vi "ConfigDlg.vi"(8 "error in (no error)":errorcluster, 11 "ScopePluginsBase in":refnum<class "ScopePluginsBase.lvclass">) -> (0 "error out":errorcluster, 3 "ScopePluginsBase out":refnum<class "ScopePluginsBase.lvclass">)   [LabVIEW 2018, in "ScopePlugins.lvlib" / "ScopePluginsBase.lvclass"]
uses:
  ScopePluginsBase.lvclass
  C:/Program Files (x86)/National Instruments/LabVIEW 2018/user.lib/NIST/BaseClasses/BasePlugin_class/BasePlugin.lvclass
  Shared/TypeDefs/Acquisition.ctl
  Shared/TypeDefs/Trigger.ctl
  Shared/TypeDefs/Channel.ctl
  TypeDefs/InitOptions.ctl
  ScopePluginsBase.lvclass/ScopePluginsBase.ctl
  Shared/TypeDefs/Channels.ctl
  <userlib>/NIST/BaseClasses/BasePlugin_class/BasePlugin.lvclass/BasePlugin.ctl
  Accessors/Read Acquisition.vi
  Accessors/Read Channels.vi
  Accessors/Read Trigger.vi
  <userlib>/NIST/BaseClasses/BasePlugin_class/Accessors/Read PluginIniFilePath.vi
  Accessors/Write Acquisition.vi
  Accessors/Write Trigger.vi
  Accessors/Write Channels.vi
  <vilib>/Utility/config.llb/NI_LVConfig.lvlib
  ScopePlugins.lvlib
panel:
  in  "Trigger Type":T1(tab)
  in  "Input Impedance":u32(ring) items=["1 mega ohm"=0, "50 ohms"=2]
  in  "Maximum Input Frequency":dbl caption="Max. Input Frequency (Hz)" format="%.2f"
  in  "Initialize Options":T2
  out "Actual Sample Rate":dbl=10000000.0 format="%#.2p"
  out "Actual Record Length":i32=1000
  in  "Min Record Length":i32=1000 caption="Min. Record Length"
  in  "Min Sample Rate":dbl=10000000.0 caption="Min. Sample Rate" step=1000000.0 format="%#.2p"
  in  "Enforce Realtime":bool=TRUE
  in  "Vertical Coupling":i32(ring)=1 items=["AC", "DC", "Ground"]
  in  "Probe Attenuation":dbl=1.0 format="%.1f"
  in  "Vertical Offset":dbl caption="Vertical Offset (V)" format="%.2p"
  in  "Vertical Range":dbl=5.0 caption="Vertical Range (V)" format="%.2f"
  in  "Trigger Type 2":T3(tab) caption="Trigger Type"
  in  "Trigger Source":string(combo)="0"
  in  "Trigger Level":dbl format="%.2f"
  in  "Trigger Slope":i32(ring) items=["Positive", "Negative"]
  in  "Coupling":u16(ring)=1 caption="Trigger Coupling" items=["AC"=0, "DC"=1, "HF Reject"=3, "LF Reject"=4, "AC Plus HF Reject"=1001]
  in  "Trigger Slope 2":i32(ring) caption="Trigger Slope" items=["Positive", "Negative"]
  in  "Trigger Source 2":string(combo)="VAL_PFI_1" caption="Trigger Source"
  in  "Coupling 2":u16(ring)=1 caption="Trigger Coupling" items=["AC"=0, "DC"=1, "HF Reject"=3, "LF Reject"=4, "AC Plus HF Reject"=1001]
  in  "High Level":dbl=0.1 caption="Window High Level" format="%.2f"
  in  "Low Level":dbl=-0.1 caption="Window Low Level" format="%.2f"
  in  "Window Mode":i32(ring) items=["Entering", "Leaving"]
  in  "Trigger Source 3":string(combo)="0" caption="Trigger Source"
  in  "Hysteresis":dbl=0.05 format="%.2f"
  in  "Trigger Source 4":string(combo)="0" caption="Trigger Source"
  in  "Trigger Level 2":dbl caption="Trigger Level" format="%.2f"
  in  "Coupling 3":u16(ring)=1 caption="Trigger Coupling" items=["AC"=0, "DC"=1, "HF Reject"=3, "LF Reject"=4, "AC Plus HF Reject"=1001]
  in  "Trigger Slope 3":i32(ring) caption="Trigger Slope" items=["Positive", "Negative"]
  out "Auto Triggered":bool
  in  "Trigger Modifier":i32(ring)=2 items=["None"=1, "Auto Trigger"=2]
  in  "Stop":bool
  in  "Reference Position":dbl=50.0 caption="Ref Position" format="%.1f"
  in  "Trigger Delay":dbl caption="Trigger Delay (s)" format="%#.4p"
  in  "InitOptions":T2
  in  "Save As Button":bool
  in  "Save Button":bool
  in  "Channels":T4[](array[typedef])
  in  "Trigger":T5
  in  "Acquisition":T6={"StartTime"=0.0, "Type"=enum."Normal", "NumPointsMin"=0, "RecordLength"=0, "SampleRate"=0.0, "TimePerRecord"=0.0, "SamplingMode "=enum."Real Time", "Interpolation"=enum."No Interpolation", "NumAverages"=8, "Resolution"=enum."Auto", "EnableAveraging"=FALSE, "Continuous"=FALSE}
  in  "btnCancel":bool
  # "Channel"
  # "Horizontal"
  # "Vertical"
  # "Trigger"
  # "Common Trigger Settings"
  # "Note: When configured for Immediate reference trigger, this example does not configure any additional trigger settings - the acquisition is triggered as soon as possible after being initiated by driver software."
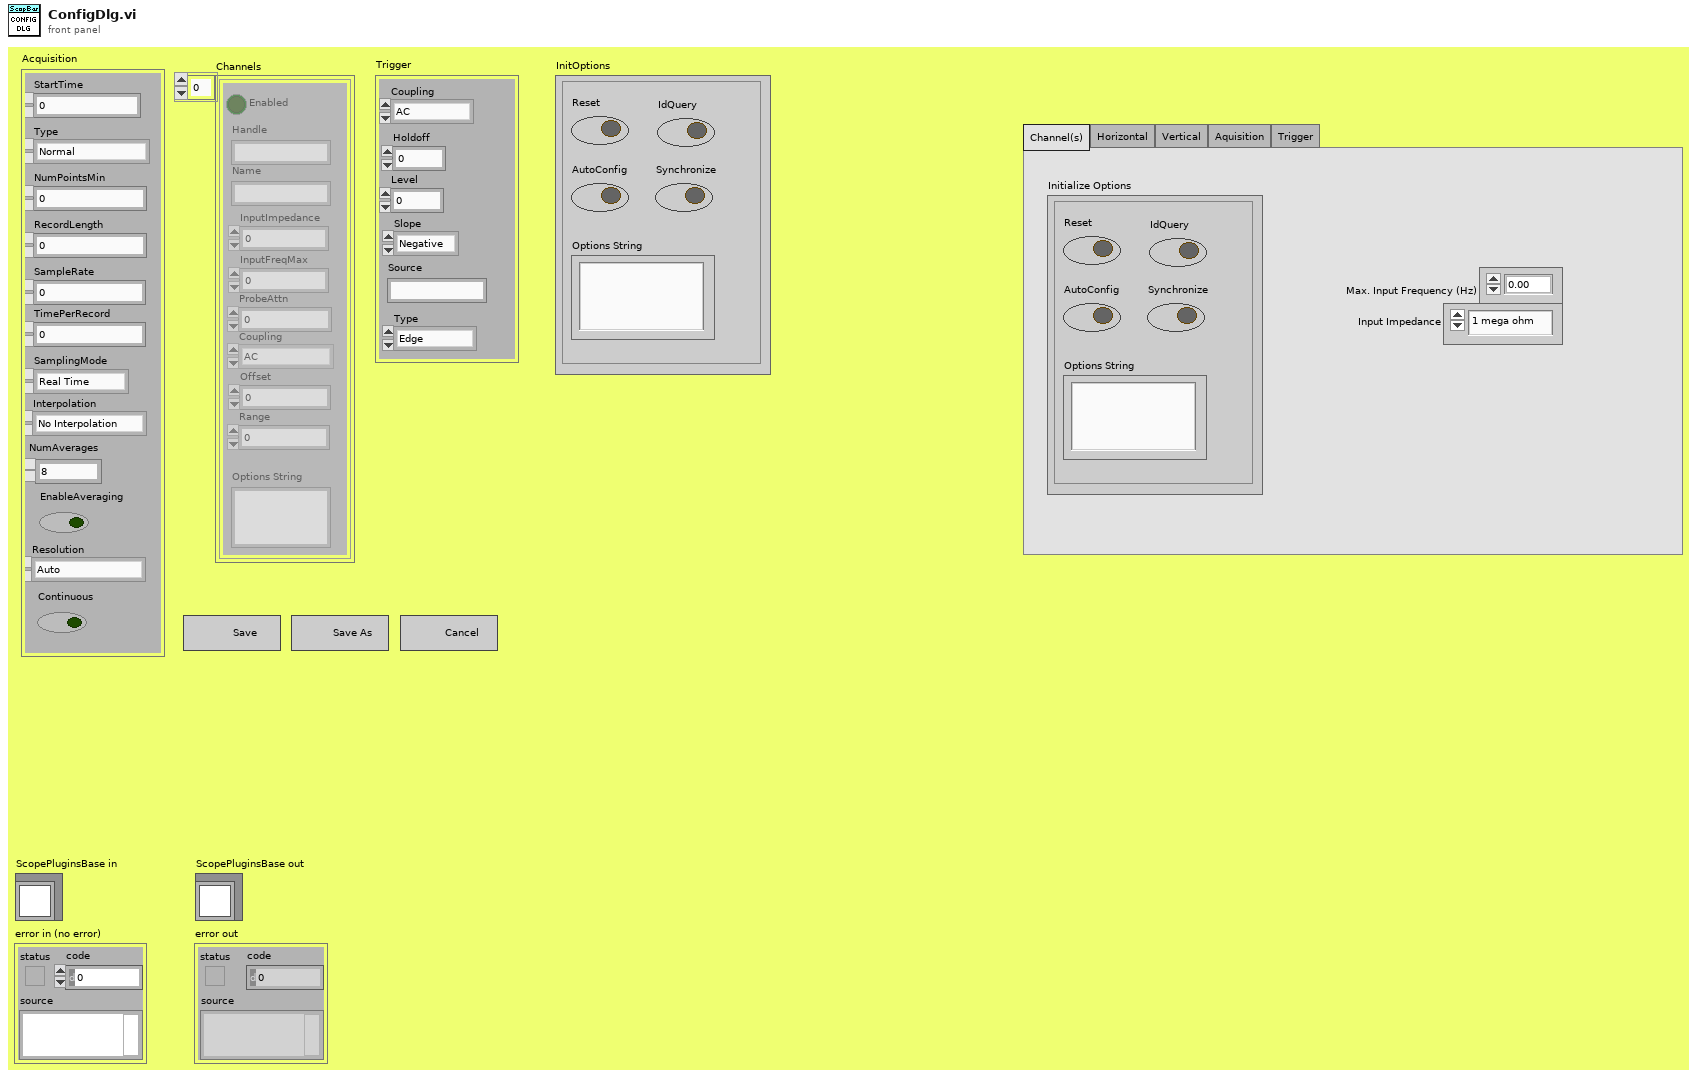
[diagram p1: front panel]
types:
  T1 = enum32{"Channel(s)", "Horizontal", "Vertical", "Aquisition", "Trigger"}
  T2 = typedef "ScopePlugins.lvlib/InitOptions.ctl" = cluster{"Reset":bool, "IdQuery":bool, "AutoConfig":bool, "Options String":string, "Synchronize":bool}
  T3 = enum32{"Immediate", "Edge", "Digital", "Window", "Hysteresis"}
  T4 = typedef "ScopePlugins.lvlib/Channel.ctl" = cluster{"Enabled":bool, "Name":string, "InputImpedance":dbl, "InputFreqMax":dbl, "ProbeAttn":dbl, "Coupling":enum16{"AC", "DC", "GND"}, "Offset":dbl, "Range":dbl, "Handle":string, "Connected":bool, "Options String ":string}
  T5 = typedef "ScopePlugins.lvlib/Trigger.ctl" = cluster{"Coupling":enum16{"AC", "DC", "LF Reject", "HF Reject", "Noise Reject"}, "Holdoff":dbl, "Level":dbl, "Slope":enum16{"Negative", "Positive"}, "Source":string, "Type":enum16{"Edge", "Width", "Runt", "Glitch", "TV", "Immediate", "AC Line"}}
  T6 = typedef "ScopePlugins.lvlib/Acquisition.ctl" = cluster{"StartTime":dbl, "Type":enum16{"Normal", "PeakDetect", "HighRes", "Envelope", "Average"}, "NumPointsMin":i32, "RecordLength":i32, "SampleRate":dbl, "TimePerRecord":dbl, "SamplingMode ":enum16{"Real Time", "Equivalent Time", "Segment", "Real Time Peak Detect", "Real Time High Resolution", "Peak Detect Segment", "High Resolution Segment"}, "Interpolation":enum16{"No Interpolation", "sin(x)/x", "linear", "1 Point sin(x)/x", "2 Point sin(x)/x", "4 Point sin(x)/x", "8 Point sin(x)/x", "16 Point sin(x)/x"}, "NumAverages":i32, "Resolution":enum16{"Auto", "Bits 9", "Bits 10", "Bits 11", "Bits 12"}, "EnableAveraging":bool, "Continuous":bool}
  T7 = enum8{"Enabled", "Disabled", "Disabled and Grayed Out"}
  T8 = enum32{"Invalid", "Default", "Floating", "Floating/Auto-Hide", "Modal"}
  T9 = typedef "ScopePlugins.lvlib/Channels.ctl" = cluster{"Count":i32, "ChannelArray":T4[]}
  T10 = typedef "NI_LVConfig.lvlib/Config Data RefNum.ctl" = refnum<k1>
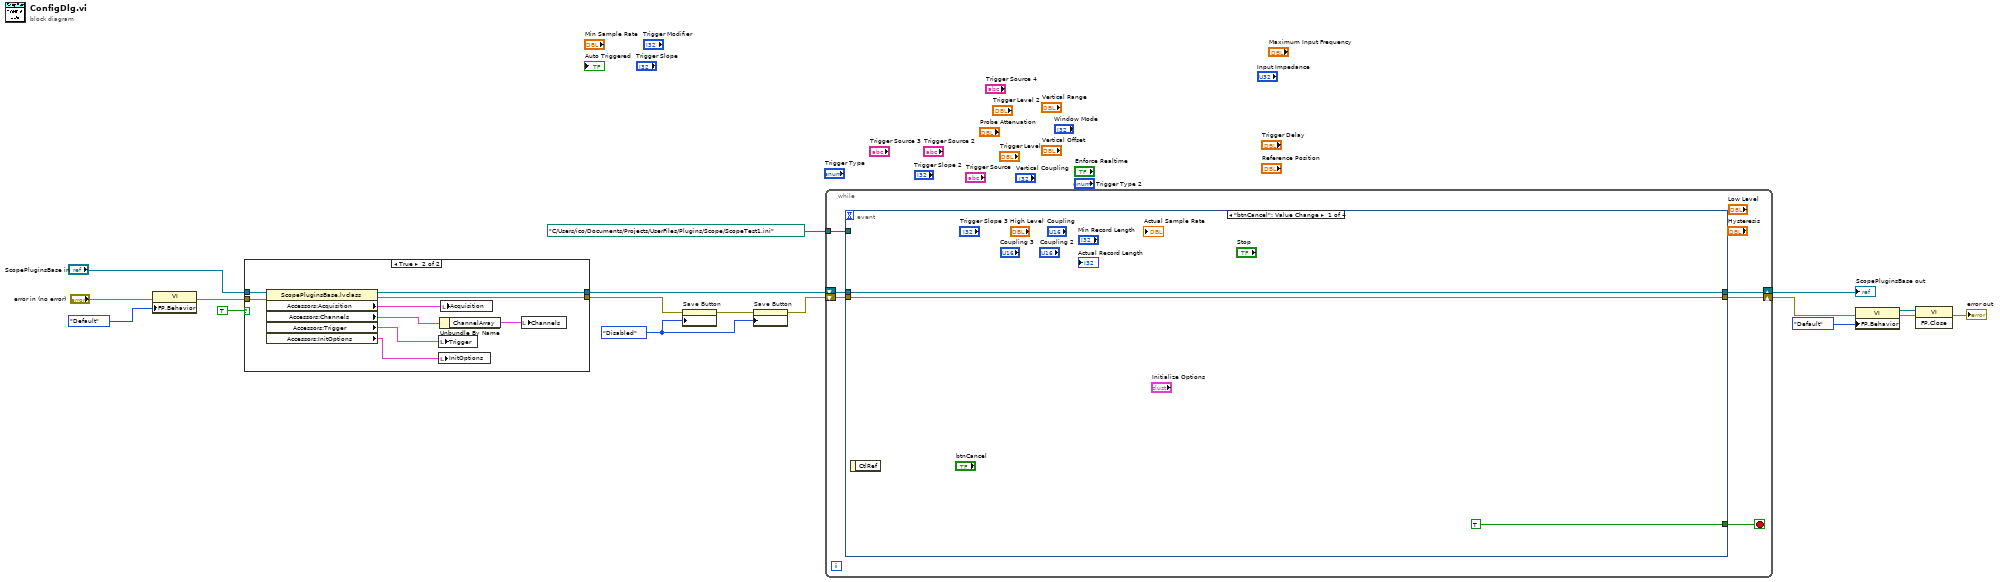
[diagram p0: block diagram]
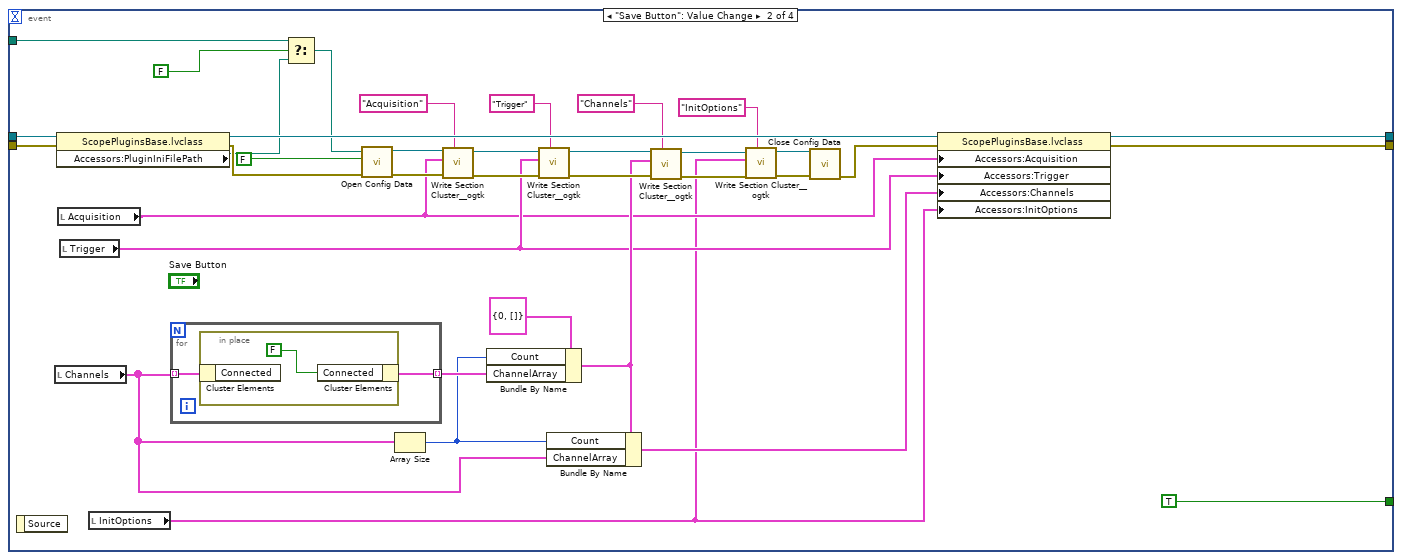
[diagram p2: hidden frame]
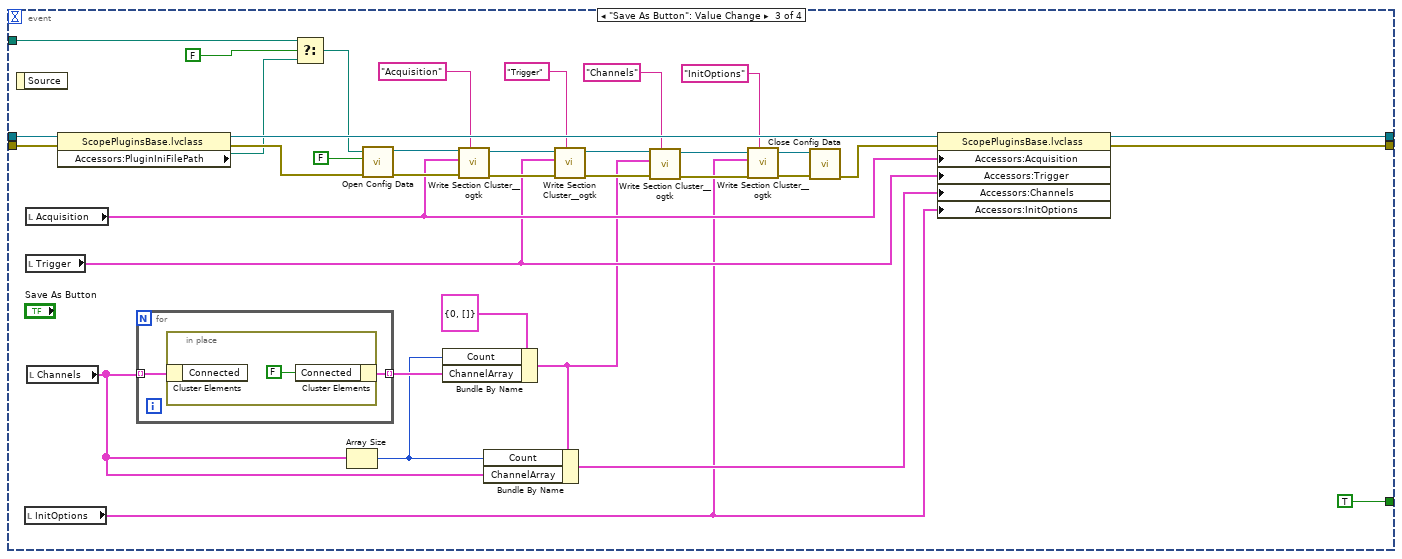
[diagram p3: hidden frame]
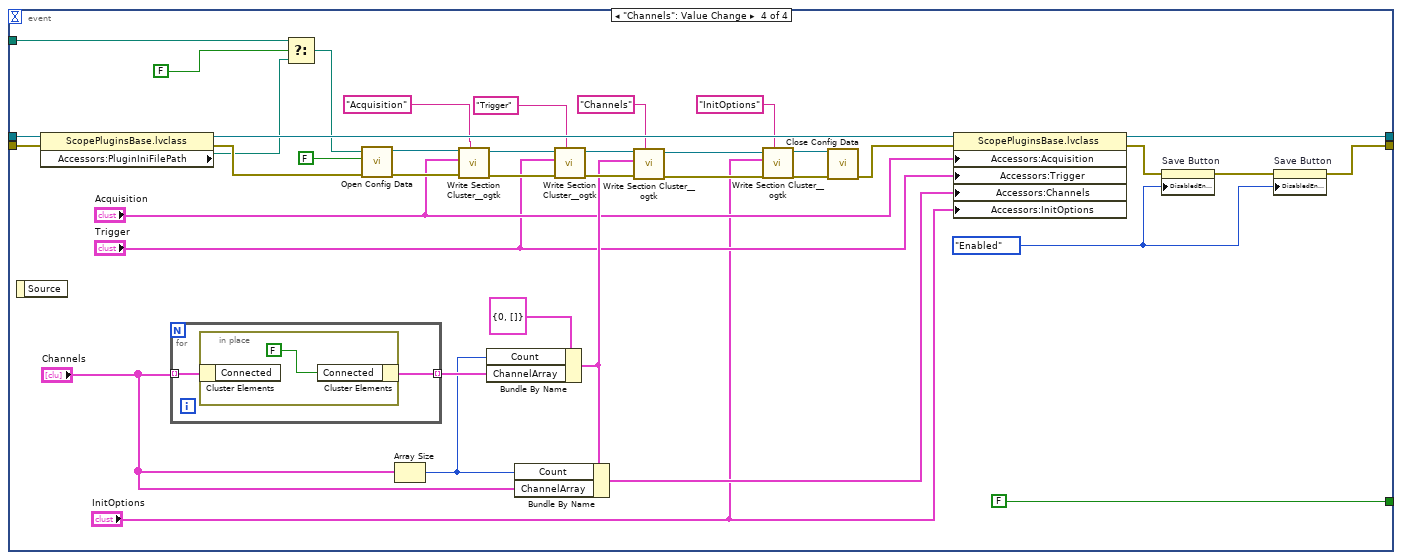
[diagram p4: hidden frame]
diagram:
  w1 = T7."Disabled" ("Disabled")
  n1 = property class="VI"(error in="error in (no error)", "FP.Behavior"=T8."Default" ("Front Panel Window:Behavior")) -> (error out=w5:errorcluster)  [unwired: 1 in, 1 out]
  n2 = case shown="True" TRUE {
    tunnel: "ScopePluginsBase in" -> [w19 w28]
    tunnel: [w19 w27] -> w16
    tunnel: w5 -> [w18 w25]
    tunnel: [w18 w21] -> w4
    frame False {
    }
    frame True {
      n3 = property class="ScopePluginsBase.lvclass"(reference=w28, error in=w25) -> (reference out=w27:refnum<class "ScopePluginsBase.lvclass">, error out=w21:errorcluster, "Accessors:Acquisition"=w24:T6, "Accessors:Channels"=w26:T9, "Accessors:Trigger"=w23:T5, "Accessors:InitOptions"=w20:T2)
      n4 = local write "InitOptions"(w20) -> ()
      n5 = local write "Trigger"(w23) -> ()
      n6 = Unbundle By Name(w26) -> ("ChannelArray"=w22:T4[])
      n7 = local write "Acquisition"(w24) -> ()
      n8 = local write "Channels"(w22) -> ()
    }
  }
  n9 = property on="Save Button" class="Bool"(error in=w4, "DisabledEnum"=w1) -> (error out=w3:errorcluster)  [unwired: 1 in, 1 out]
  n10 = property on="Save Button" class="Bool"(error in=w3, "DisabledEnum"=w1) -> (error out=w2:errorcluster)  [unwired: 1 in, 1 out]
  n11 = while {
    tunnel: path "C:/Users/ico/Documents/Projects/UserFiles/Plugins/Scope/ScopeTest1.ini" ("PluginIniFilePath") -> [w30]
    shift-right: [w33] -> w15
    shift-left: w16 -> [w34]
    shift-right: [w32] -> w13
    shift-left: w2 -> [w31]
    stop <- w29 stop-if-true
    n12 = event shown="[0] \"btnCancel\": Value Change" {
      selector: _ -> [_ _ _ _]
      dyn-events: _ -> [_ _ _ _]
      timeout: _ -> [_ _ _ _]
      tunnel: w31 -> [w37 w72 w111 w153]
      tunnel: [w37 w61 w100 w124] -> w32
      tunnel: w34 -> [w36 w73 w112 w154]
      tunnel: [w36 w62 w101 w143] -> w33
      tunnel: w30 -> [_ w52 w91 w134]
      tunnel: [TRUE ("stop") TRUE ("stop") TRUE ("stop") FALSE ("stop")] -> w29
      event "btnCancel": Value Change {
        n13 = event-data() -> ()  [unwired: 1 in, 1 out]
      }
      event "Save Button": Value Change {
        n14 = event-data() -> ()  [unwired: 1 in, 1 out]
        n15 = local read "Channels"() -> (w48:T4[])
        n16 = property class="ScopePluginsBase.lvclass"(reference=w73, error in=w72) -> (reference out=w60:refnum<class "ScopePluginsBase.lvclass">, error out=w67:errorcluster, "Accessors:PluginIniFilePath"=w54:path)
        n17 = local read "Acquisition"() -> (w46:T6)
        n18 = local read "Trigger"() -> (w47:T5)
        n19 = local read "InitOptions"() -> (w38:T2)
        n20 = for {
          tunnel: [w75] -> w56 mode=indexing
          tunnel: w48 -> [w74] mode=indexing
          n21 = in-place {
            n22 = in-place-cluster #1(w74) -> ()  [unwired: 1 out]
            n23 = in-place-cluster #1("Connected"=FALSE) -> (w75:T4)
          }
        }
        n24 = Select(t=w52, s=FALSE, f=w54) -> (s? t:f=w53:path)
        n25 = call <vilib>:"Open Config Data.vi"("error in (no error)"=w67, "create file if necessary (T)"=FALSE, "configuration file path"=w53) -> ("error out"=w70:errorcluster, "refnum"=w71:T10)  [unwired: 6 in, 1 out]
        n26 = Array Size(array=w48) -> (size(s)=w55:i32)
        n27 = call <userlib>:"Write Section Cluster__ogtk.vi"("section (optional)"="Acquisition", "error in (no error)"=w70, "Section Formatted Cluster"=w46, "refnum"=w71) -> ("error out"=w69:errorcluster, "dup refnum"=w65:T10)  [unwired: 6 in]
        n28 = Bundle By Name(cluster=T9 {"Count"=0, "ChannelArray"=[]} ("Channels"), "Count"=w55, "ChannelArray"=w56) -> (w49:T9)
        n29 = call <userlib>:"Write Section Cluster__ogtk.vi"("section (optional)"="Trigger", "error in (no error)"=w69, "Section Formatted Cluster"=w47, "refnum"=w65) -> ("error out"=w66:errorcluster, "dup refnum"=w64:T10)  [unwired: 6 in]
        n30 = Bundle By Name(cluster=w49, "Count"=w55, "ChannelArray"=w48) -> (w58:T9)
        n31 = call <userlib>:"Write Section Cluster__ogtk.vi"("section (optional)"="Channels", "error in (no error)"=w66, "Section Formatted Cluster"=w49, "refnum"=w64) -> ("error out"=w42:errorcluster, "dup refnum"=w41:T10)  [unwired: 6 in]
        n32 = call <userlib>:"Write Section Cluster__ogtk.vi"("section (optional)"="InitOptions", "error in (no error)"=w42, "Section Formatted Cluster"=w38, "refnum"=w41) -> ("error out"=w40:errorcluster, "dup refnum"=w39:T10)  [unwired: 6 in]
        n33 = call <vilib>:"Close Config Data.vi"("error in (no error)"=w40, "refnum"=w39) -> ("error out"=w63:errorcluster)  [unwired: 8 in, 1 out]
        n34 = property class="ScopePluginsBase.lvclass"(reference=w60, error in=w63, "Accessors:Acquisition"=w46, "Accessors:Trigger"=w47, "Accessors:Channels"=w58, "Accessors:InitOptions"=w38) -> (reference out=w62:refnum<class "ScopePluginsBase.lvclass">, error out=w61:errorcluster)
      }
      event "Save As Button": Value Change {
        n35 = event-data() -> ()  [unwired: 1 in, 1 out]
        n36 = local read "InitOptions"() -> (w77:T2)
        n37 = local read "Acquisition"() -> (w88:T6)
        n38 = local read "Trigger"() -> (w87:T5)
        n39 = local read "Channels"() -> (w85:T4[])
        n40 = property class="ScopePluginsBase.lvclass"(reference=w112, error in=w111) -> (reference out=w99:refnum<class "ScopePluginsBase.lvclass">, error out=w106:errorcluster, "Accessors:PluginIniFilePath"=w93:path)
        n41 = for {
          tunnel: [w114] -> w95 mode=indexing
          tunnel: w85 -> [w113] mode=indexing
          n42 = in-place {
            n43 = in-place-cluster #2(w113) -> ()  [unwired: 1 out]
            n44 = in-place-cluster #2("Connected"=FALSE) -> (w114:T4)
          }
        }
        n45 = Select(t=w91, s=FALSE, f=w93) -> (s? t:f=w92:path)
        n46 = Array Size(array=w85) -> (size(s)=w94:i32)
        n47 = call <vilib>:"Open Config Data.vi"("error in (no error)"=w106, "create file if necessary (T)"=FALSE, "configuration file path"=w92) -> ("error out"=w109:errorcluster, "refnum"=w110:T10)  [unwired: 6 in, 1 out]
        n48 = Bundle By Name(cluster=T9 {"Count"=0, "ChannelArray"=[]} ("Channels"), "Count"=w94, "ChannelArray"=w95) -> (w86:T9)
        n49 = call <userlib>:"Write Section Cluster__ogtk.vi"("section (optional)"="Acquisition", "error in (no error)"=w109, "Section Formatted Cluster"=w88, "refnum"=w110) -> ("error out"=w108:errorcluster, "dup refnum"=w104:T10)  [unwired: 6 in]
        n50 = Bundle By Name(cluster=w86, "Count"=w94, "ChannelArray"=w85) -> (w97:T9)
        n51 = call <userlib>:"Write Section Cluster__ogtk.vi"("section (optional)"="Trigger", "error in (no error)"=w108, "Section Formatted Cluster"=w87, "refnum"=w104) -> ("error out"=w105:errorcluster, "dup refnum"=w103:T10)  [unwired: 6 in]
        n52 = call <userlib>:"Write Section Cluster__ogtk.vi"("section (optional)"="Channels", "error in (no error)"=w105, "Section Formatted Cluster"=w86, "refnum"=w103) -> ("error out"=w82:errorcluster, "dup refnum"=w81:T10)  [unwired: 6 in]
        n53 = call <userlib>:"Write Section Cluster__ogtk.vi"("section (optional)"="InitOptions", "error in (no error)"=w82, "Section Formatted Cluster"=w77, "refnum"=w81) -> ("error out"=w80:errorcluster, "dup refnum"=w79:T10)  [unwired: 6 in]
        n54 = call <vilib>:"Close Config Data.vi"("error in (no error)"=w80, "refnum"=w79) -> ("error out"=w102:errorcluster)  [unwired: 8 in, 1 out]
        n55 = property class="ScopePluginsBase.lvclass"(reference=w99, error in=w102, "Accessors:Acquisition"=w88, "Accessors:Trigger"=w87, "Accessors:Channels"=w97, "Accessors:InitOptions"=w77) -> (reference out=w101:refnum<class "ScopePluginsBase.lvclass">, error out=w100:errorcluster)
      }
      event "Channels": Value Change {
        w126 = T7."Enabled" ("Disabled")
        n56 = event-data() -> ()  [unwired: 1 in, 1 out]
        n57 = property class="ScopePluginsBase.lvclass"(reference=w154, error in=w153) -> (reference out=w142:refnum<class "ScopePluginsBase.lvclass">, error out=w148:errorcluster, "Accessors:PluginIniFilePath"=w136:path)
        n58 = for {
          tunnel: [w156] -> w138 mode=indexing
          tunnel: "Channels" -> [w155] mode=indexing
          n59 = in-place {
            n60 = in-place-cluster #3(w155) -> ()  [unwired: 1 out]
            n61 = in-place-cluster #3("Connected"=FALSE) -> (w156:T4)
          }
        }
        n62 = Select(t=w134, s=FALSE, f=w136) -> (s? t:f=w135:path)
        n63 = call <vilib>:"Open Config Data.vi"("error in (no error)"=w148, "create file if necessary (T)"=FALSE, "configuration file path"=w135) -> ("error out"=w151:errorcluster, "refnum"=w152:T10)  [unwired: 6 in, 1 out]
        n64 = Array Size(array="Channels") -> (size(s)=w137:i32)
        n65 = call <userlib>:"Write Section Cluster__ogtk.vi"("section (optional)"="Acquisition", "error in (no error)"=w151, "Section Formatted Cluster"="Acquisition", "refnum"=w152) -> ("error out"=w150:errorcluster, "dup refnum"=w146:T10)  [unwired: 6 in]
        n66 = Bundle By Name(cluster=T9 {"Count"=0, "ChannelArray"=[]} ("Channels"), "Count"=w137, "ChannelArray"=w138) -> (w131:T9)
        n67 = Bundle By Name(cluster=w131, "Count"=w137, "ChannelArray"="Channels") -> (w140:T9)
        n68 = call <userlib>:"Write Section Cluster__ogtk.vi"("section (optional)"="Trigger", "error in (no error)"=w150, "Section Formatted Cluster"="Trigger", "refnum"=w146) -> ("error out"=w147:errorcluster, "dup refnum"=w145:T10)  [unwired: 6 in]
        n69 = call <userlib>:"Write Section Cluster__ogtk.vi"("section (optional)"="Channels", "error in (no error)"=w147, "Section Formatted Cluster"=w131, "refnum"=w145) -> ("error out"=w120:errorcluster, "dup refnum"=w119:T10)  [unwired: 6 in]
        n70 = call <userlib>:"Write Section Cluster__ogtk.vi"("section (optional)"="InitOptions", "error in (no error)"=w120, "Section Formatted Cluster"="InitOptions", "refnum"=w119) -> ("error out"=w117:errorcluster, "dup refnum"=w118:T10)  [unwired: 6 in]
        n71 = call <vilib>:"Close Config Data.vi"("error in (no error)"=w117, "refnum"=w118) -> ("error out"=w144:errorcluster)  [unwired: 8 in, 1 out]
        n72 = property class="ScopePluginsBase.lvclass"(reference=w142, error in=w144, "Accessors:Acquisition"="Acquisition", "Accessors:Trigger"="Trigger", "Accessors:Channels"=w140, "Accessors:InitOptions"="InitOptions") -> (reference out=w143:refnum<class "ScopePluginsBase.lvclass">, error out=w125:errorcluster)
        n73 = property on="Save Button" class="Bool"(error in=w125, "DisabledEnum"=w126) -> (error out=w127:errorcluster)  [unwired: 1 in, 1 out]
        n74 = property on="Save Button" class="Bool"(error in=w127, "DisabledEnum"=w126) -> (error out=w124:errorcluster)  [unwired: 1 in, 1 out]
      }
    }
  }
  "ScopePluginsBase out" <- w15
  n75 = property class="VI"(error in=w13, "FP.Behavior"=T8."Default" ("Front Panel Window:Behavior")) -> (reference out=w14:refnum<vi>, error out=w12:errorcluster)  [unwired: 1 in]
  n76 = invoke class="VI" method="FP.Close"(reference=w14, error in=w12) -> (error out=→"error out":errorcluster)  [unwired: 1 in, 2 out]
